vi "thermometer.vi"(9 "lower bound value":dbl, 11 "upper bound value":dbl) -> (3 "random degC":dbl)   [LabVIEW 2014]
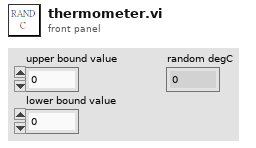
[diagram p1: front panel]
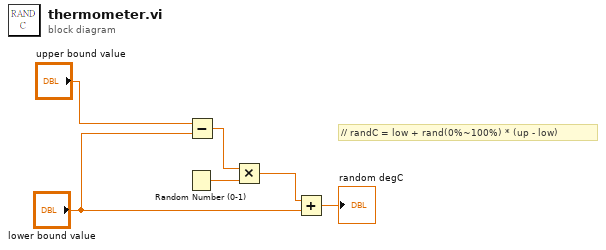
[diagram p0: block diagram]
diagram:
  # "// randC = low + rand(0%~100%) * (up - low)"
  n1 = Random Number (0-1)() -> (number: 0 to 1=w4:dbl)
  n2 = Subtract(x="upper bound value", y="lower bound value") -> (x-y=w5:dbl)
  n3 = Multiply(x=w5, y=w4) -> (x*y=w2:dbl)
  n4 = Add(x=w2, y="lower bound value") -> (x+y=→"random degC":dbl)
